vi "basic_encoder.vi"(8 "error in (no error)":errorcluster, 11 "Test Data in":T1) -> (0 "error out":errorcluster, 3 "Test Data out":T1)   [LabVIEW 2024, in "Tester.lvlib"]
uses:
  Tester.lvlib
  test_data--cluster.ctl
  packetized_data--cluster.ctl
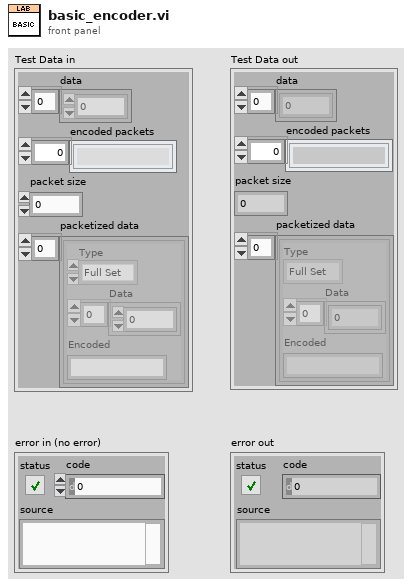
[diagram p1: front panel]
types:
  T1 = typedef "Tester.lvlib/test_data--cluster.ctl" = cluster{"data":dbl[], "encoded packets":string[], "packet size":i32, "packetized data":T2[]}
  T2 = typedef "Tester.lvlib/packetized_data--cluster.ctl" = cluster{"Type":enum16{"Full Set", "Last Set"}, "Data":dbl[], "Encoded":string}
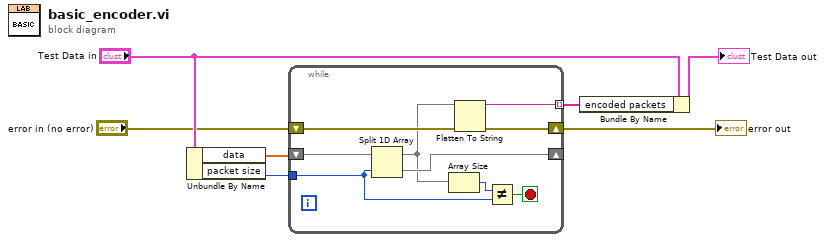
[diagram p0: block diagram]
diagram:
  n1 = Unbundle By Name("Test Data in") -> ("data"=w7:dbl[], "packet size"=w6:i32)
  n2 = while {
    tunnel: w6 -> [w10]
    tunnel: [w13] -> w5 mode=indexing
    shift-right: [w12] -> w1
    shift-left: "error in (no error)" -> [w11]
    shift-right: [w9] -> _
    shift-left: w7 -> [w16]
    stop <- w14 stop-if-true
    n3 = Split 1D Array(array=w16, index=w10) -> (first subarray=w8:dbl[], second subarray=w9:dbl[])
    n4 = Array Size(array=w8) -> (size(s)=w15:i32)
    n5 = Flatten To String(anything=w8, error in (no error)=w11) -> (data string=w13:string, error out=w12:errorcluster)  [unwired: 2 in, 1 out]
    n6 = Not Equal?(x=w15, y=w10) -> (x != y?=w14:bool)
  }
  "error out" <- w1
  n7 = Bundle By Name(cluster="Test Data in", "encoded packets"=w5) -> (→"Test Data out":T1)
